vi "合格状态.vi"(7 "枚举":enum16{"Read", "Write"}(ring), 10 "工位":enum16{"工位1", "工位2", "工位3"}(ring), 11 "Status_Write":i16) -> (3 "Status_Read":i16)   [LabVIEW 2020]
uses:
  Libraries/S7/S7.lvlib
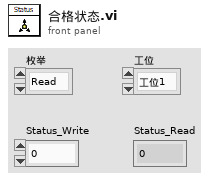
[diagram p1: front panel]
types:
  T1 = typedef "S7.lvlib/Read_Data (Reply Payload)--cluster.ctl" = cluster{"读取成功":bool, "数据":u32[], "Read_Data_error":errorcluster}
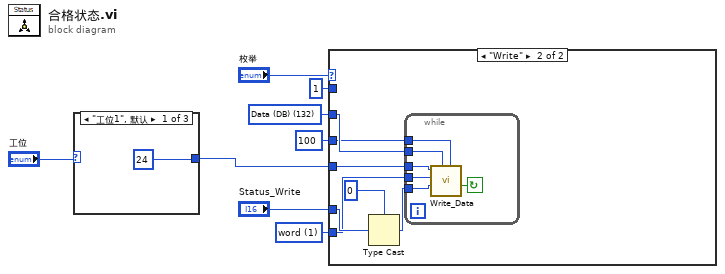
[diagram p0: block diagram]
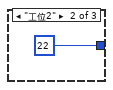
[diagram p2: hidden frame]
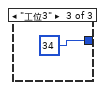
[diagram p3: hidden frame]
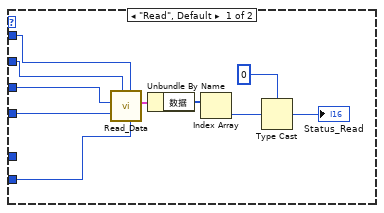
[diagram p4: hidden frame]
diagram:
  w4 = u16 1 items=["byte", "word", "Dword"] ("数据类型")
  w5 = u8 132 items=["I/O (P)"=128, "Input (I)"=129, "Output (Q)"=130, "Bit Memory (M)"=131, "Data (DB)"=132, "Instance Data (DI)"=133, "Local Data (L)"=134, "Predecessor Local Data (VL)"=135] ("寄存器类型")
  n1 = case shown="\"工位1\", 默认" "工位" {
    tunnel: [u16 24 ("DB #") u32 22 ("起始地址") u16 34] -> w3
    frame "工位1", Default {
    }
    frame "工位2" {
    }
    frame "工位3" {
    }
  }
  n2 = case shown="\"Write\"" "枚举" {
    tunnel: u16 100 ("DB #") -> [w21 w23]
    tunnel: w3 -> [w20 w22]
    tunnel: w5 -> [w19 w25]
    tunnel: u16 1 ("读取长度") -> [w18 _]
    tunnel: w4 -> [w17 w24]
    tunnel: "Status_Write" -> [_ w26]
    frame "Read", Default {
      n3 = call "Read_Data.vi"("数据类型"=w17, "读取长度"=w18, "寄存器类型"=w19, "起始地址"=w20, "DB #"=w21) -> ("Reply Payload"=w15:T1)  [unwired: 4 in, 2 out]
      n4 = Unbundle By Name(w15) -> ("数据"=w14:u32[])
      n5 = Index Array(array=w14) -> (element=w12:u32)  [unwired: 1 in]
      n6 = Type Cast(type=u32 0, x=w12) -> (*(type *) &x=→"Status_Read":u32)
    }
    frame "Write" {
      n7 = Type Cast(type=u16 0, x=w26) -> (*(type *) &x=w27:u16)
      n8 = while {
        tunnel: w27 -> [w34]
        tunnel: w25 -> [w33]
        tunnel: w24 -> [w32]
        tunnel: w23 -> [w31]
        tunnel: w22 -> [w30]
        stop <- w29 continue-if-true
        n9 = call "Write_Data.vi"("DB #"=w31, "寄存器类型"=w33, "写入数据"=w34, "数据类型"=w32, "写入地址"=w30) -> ("timed out?"=w29:bool)  [unwired: 4 in, 2 out]
      }
    }
  }
